vi "Get IOconfig wrapper.vi"(8 "error in (no error)":errorcluster caption="错误输入（无错误）", 9 "pDummyIOCInfo":T1, 10 "dwCanNodeId":u32, 11 "dwDevIndex":u32) -> (0 "error out":errorcluster caption="错误输出", 1 "pDummyIOCInfo out":T1, 3 "function return":u32)   [LabVIEW 2016, in "UISimCanFunc_wrapper.lvlib"]
doc: "_declspec (dllexport) DWORD GetIOconfig_wrapper(DWORD dwDevIndex, DWORD dwCanNodeId, P_DUMMY_IOC_INFO_OBJ pDummyIOCInfo);"
uses:
  <userlib>/UISimCanFunc_wrapper/UISimCanFunc_wrapper.lvlib
  <userlib>/UISimCanFunc_wrapper/UISimCanFunc_wrapper.dll
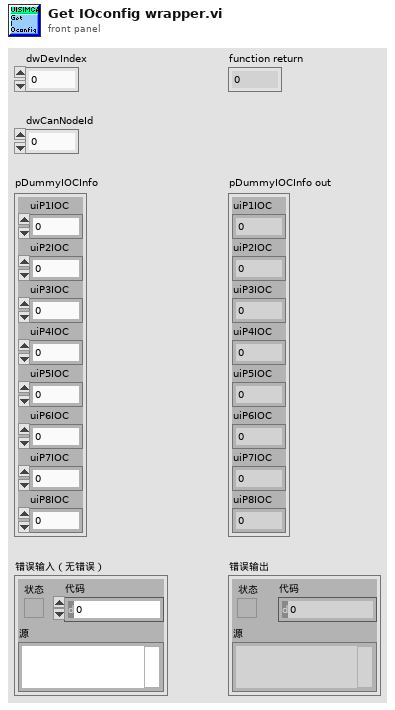
[diagram p1: front panel]
types:
  T1 = cluster{"uiP1IOC":u8, "uiP2IOC":u8, "uiP3IOC":u8, "uiP4IOC":u8, "uiP5IOC":u8, "uiP6IOC":u8, "uiP7IOC":u8, "uiP8IOC":u8}
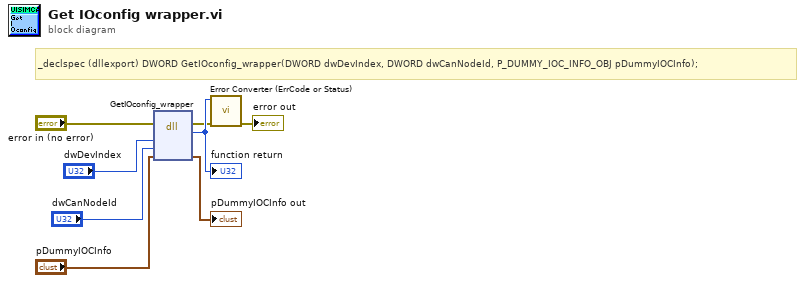
[diagram p0: block diagram]
diagram:
  # "_declspec (dllexport) DWORD GetIOconfig_wrapper(DWORD dwDevIndex, DWORD dwCanNodeId, P_DUMMY_IOC_INFO_OBJ pDummyIOCInfo);"
  n1 = dll-call lib="C:/Program Files (x86)/National Instruments/LabVIEW 2016/user.lib/UISimCanFunc_wrapper/UISimCanFunc_wrapper.*" fn="GetIOconfig_wrapper"(error in="error in (no error)", "dwDevIndex"="dwDevIndex", "dwCanNodeId"="dwCanNodeId", "pDummyIOCInfo"="pDummyIOCInfo") -> (error out=w2:errorcluster, w8:u32, "pDummyIOCInfo"=→"pDummyIOCInfo out":T1)  [unwired: 4 in, 1 out]
  "function return" <- w8
  n2 = call <userlib>:"Error Converter (ErrCode or Status).vi"("error in (no error)"=w2, "error code"=w8) -> ("error out"=→"error out":errorcluster)  [unwired: 9 in]
